vi "File Append Data to FA File.vi"(0 "error in (no error)":errorcluster, 2 "Data":dbl[][](array[numeric]), 3 "FA File Reference":refnum<file>) -> (7 "error out":errorcluster, 10 "FA File Reference":refnum<file>)   [LabVIEW 2011, in "File VIs.lvlib"]
uses:
  File VIs.lvlib
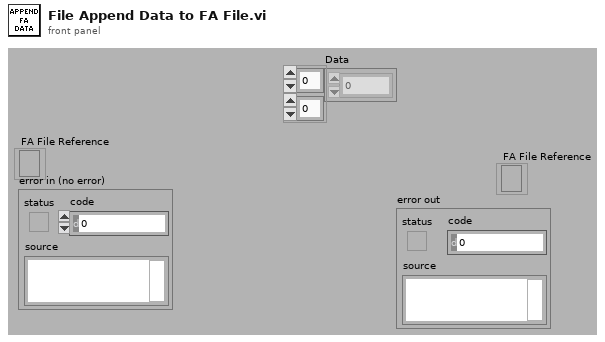
[diagram p1: front panel]
types:
  T1 = enum16{"big-endian, network order", "native, host order", "little-endian"}
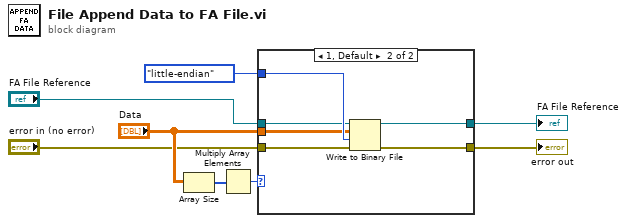
[diagram p0: block diagram]
diagram:
  n1 = Array Size(array="Data") -> (size(s)=w2:i32[])
  n2 = Multiply Array Elements(1:w2) -> (0:w1:i32)
  n3 = case shown="1, Default" w1 {
    tunnel: T1."little-endian" ("byte order (0:big-endian, network order)") -> [_ w16]
    tunnel: [w10 w15] -> w4
    tunnel: [w9 w14] -> w3
    tunnel: "FA File Reference" -> [w10 w13]
    tunnel: "error in (no error)" -> [w9 w12]
    tunnel: "Data" -> [_ w11]
    frame 0 {
    }
    frame 1, Default {
      n4 = Write to Binary File(file (use dialog)=w13, data=w11, error in=w12, 9:w16) -> (refnum out=w15:refnum<file>, error out=w14:errorcluster)  [unwired: 2 in, 1 out]
    }
  }
  "error out" <- w3
  "FA File Reference" <- w4
